vi "Get RetrContextFuncName.vi"(11 "RetrieveContextFuncName in":string caption="Embedding Model URL in") -> (3 "RetrieveContextFuncName out":string)   [LabVIEW 2023, in "LabVIEW RAG.lvlib"]
uses:
  LabVIEW RAG.lvlib
  AI RAG Globals.vi
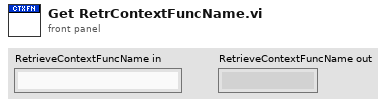
[diagram p1: front panel]
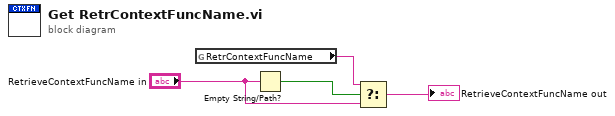
[diagram p0: block diagram]
diagram:
  n1 = global read "AI RAG Globals.vi" "RetrContextFuncName"() -> (w4:string)
  n2 = Empty String/Path?(string/path="RetrieveContextFuncName in") -> (empty?=w3:bool)
  n3 = Select(t=w4, s=w3, f="RetrieveContextFuncName in") -> (s? t:f=→"RetrieveContextFuncName out":string)
